vi "BMP180 Pull Raw Measurement.vi"(6 "Sensor Type":enum16{"Temp", "Pressure"}(ring), 8 "error in (no error)":errorcluster, 9 "BMP180 Config":T7={"I2C"={"Slave Address"=64, "Channel"=0}, "Mode"=enum."Ultra Low Power", "Cal Coefs"={"AC1"={"Addr:"=0, "Val:"=0}, "AC2"={"Addr:"=0, "Val:"=0}, "AC3"={"Addr:"=0, "Val:"=0}, "AC4"={"Addr:"=0, "Val:"=0}, "AC5"={"Addr:"=0, "Val:"=0}, "AC6"={"Addr:"=0, "Val:"=0}, "B1"={"Addr:"=0, "Val:"=0}, "B2"={"Addr:"=0, "Val:"=0}, "MB"={"Addr:"=0, "Val:"=0}, "MC"={"Addr:"=0, "Val:"=0}, "MD"={"Addr:"=0, "Val:"=0}}, "Online"=FALSE} {"I2C"."Slave Address" format="%.0x"; "Cal Coefs"."MD"."Val:" format="%04x"; "Cal Coefs"."MD"."Addr:" format="%02x"; "Cal Coefs"."MC"."Val:" format="%04x"; "Cal Coefs"."MC"."Addr:" format="%02x"; "Cal Coefs"."MB"."Val:" format="%04x"; "Cal Coefs"."MB"."Addr:" format="%02x"; "Cal Coefs"."B2"."Val:" format="%04x"; "Cal Coefs"."B2"."Addr:" format="%02x"; "Cal Coefs"."B1"."Val:" format="%04x"; "Cal Coefs"."B1"."Addr:" format="%02x"; "Cal Coefs"."AC6"."Val:" format="%04x"; "Cal Coefs"."AC6"."Addr:" format="%02x"; "Cal Coefs"."AC5"."Val:" format="%04x"; "Cal Coefs"."AC5"."Addr:" format="%02x"; "Cal Coefs"."AC4"."Val:" format="%04x"; "Cal Coefs"."AC4"."Addr:" format="%02x"; "Cal Coefs"."AC3"."Val:" format="%04x"; "Cal Coefs"."AC3"."Addr:" format="%02x"; "Cal Coefs"."AC2"."Val:" format="%04x"; "Cal Coefs"."AC2"."Addr:" format="%02x"; "Cal Coefs"."AC1"."Val:" format="%04x"; "Cal Coefs"."AC1"."Addr:" format="%02x"}, 11 "LINX Resource in":T1) -> (0 "error out":errorcluster, 2 "Raw Reading":i32, 3 "LINX Resource":T1)   [LabVIEW 2017]
uses:
  BMP180 Config Options.ctl
  <vilib>/MakerHub/LINX/Private/Type Defs/LINX Ref.ctl
  <vilib>/MakerHub/LINX/Private/Type Defs/Platform.ctl
  <vilib>/MakerHub/LINX/Private/Type Defs/Interface.ctl
  <vilib>/MakerHub/LINX/Private/Device/Type Defs/LINX Device Config.ctl
  <vilib>/MakerHub/LINX/Private/Device/Type Defs/TCP Config.ctl
  <vilib>/MakerHub/LINX/Private/Device/Type Defs/Channels.ctl
  <vilib>/MakerHub/LINX/LMH-LINX.lvlib
  <vilib>/MakerHub/LINX/Private/Device/Device.lvlib
panel:
  out "Data":u8[](array[numeric]) format="%.0x"
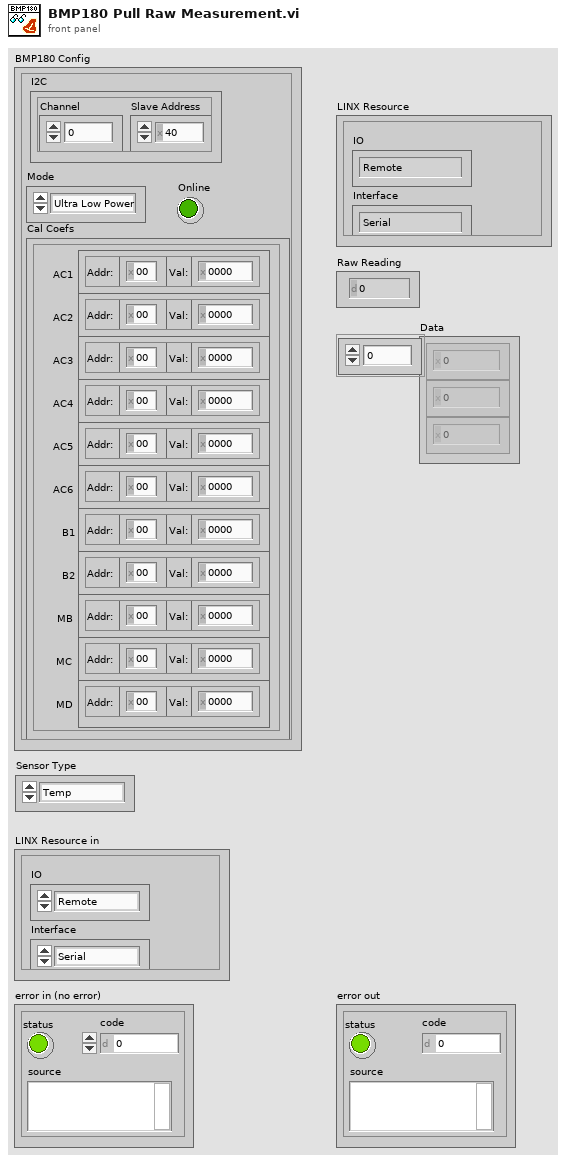
[diagram p1: front panel]
types:
  T1 = typedef "LMH-LINX.lvlib/LINX Ref.ctl" = cluster{"IO":T2, "Interface":T3, "LINX Device Config":T4}
  T2 = typedef "LMH-LINX.lvlib/Platform.ctl" = enum16{"Remote", "Local"}
  T3 = typedef "LMH-LINX.lvlib/Interface.ctl" = enum16{"Serial", "TCP"}
  T4 = typedef "LMH-LINX.lvlib/Device.lvlib/LINX Device Config.ctl" = cluster{"Interface":T3, "COM Port":refnum<visa-resource-name>, "TCP Configuration":T5, "Device Family":u8, "Device ID":u8, "Device Name":string, "TCP Ref":refnum<k5>, "Channels":T6}
  T5 = typedef "LMH-LINX.lvlib/Device.lvlib/TCP Config.ctl" = cluster{"IP Address":string, "Port":u16}
  T6 = typedef "LMH-LINX.lvlib/Channels.ctl" = cluster{"DI":u8[], "DO":u8[], "AI":u8[], "AO":u8[], "PWM":u8[], "QE":u8[], "UART":u8[], "I2C 2":u8[], "SPI":u8[], "CAN":u8[], "Servo":u8[], "AI Ref (V)":dbl, "AI Resolution (Bits)":u8, "AO Ref (V)":dbl, "AO Resolution (Bits)":u8}
  T7 = typedef "BMP180 Config Options.ctl" = cluster{"I2C":cluster{"Slave Address":u8, "Channel":u8}, "Mode":enum8{"Ultra Low Power", "Standard", "High Resolution", "Ultra High Resolution"}, "Cal Coefs":cluster{"AC1":cluster{"Addr:":u8, "Val:":u16}, "AC2":cluster{"Addr:":u8, "Val:":u16}, "AC3":cluster{"Addr:":u8, "Val:":u16}, "AC4":cluster{"Addr:":u8, "Val:":u16}, "AC5":cluster{"Addr:":u8, "Val:":u16}, "AC6":cluster{"Addr:":u8, "Val:":u16}, "B1":cluster{"Addr:":u8, "Val:":u16}, "B2":cluster{"Addr:":u8, "Val:":u16}, "MB":cluster{"Addr:":u8, "Val:":u16}, "MC":cluster{"Addr:":u8, "Val:":u16}, "MD":cluster{"Addr:":u8, "Val:":u16}}, "Online":bool}
  T8 = enum8{"Ultra Low Power", "Standard", "High Resolution", "Ultra High Resolution"}
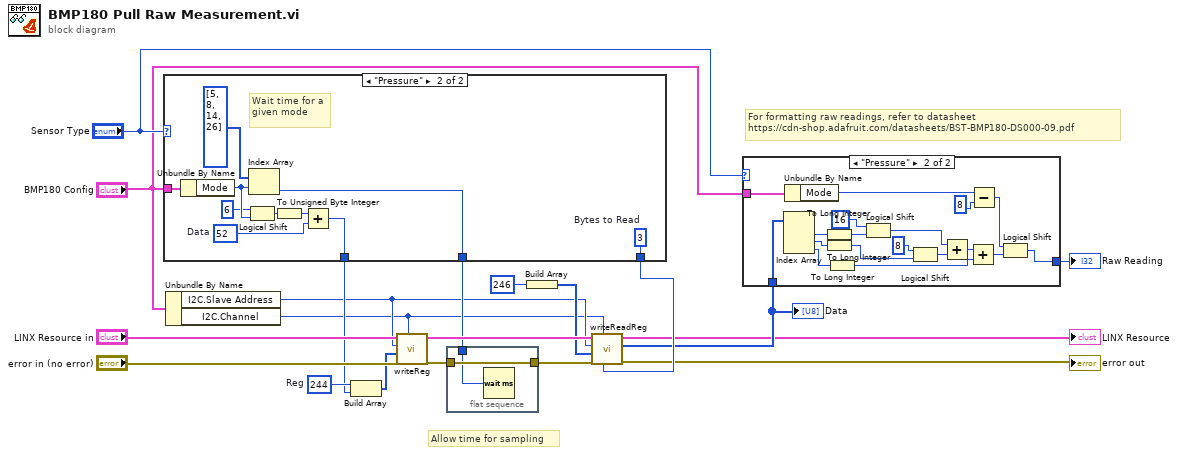
[diagram p0: block diagram]
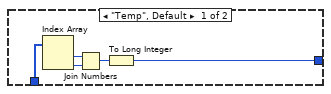
[diagram p2: hidden frame]
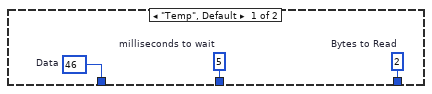
[diagram p3: hidden frame]
diagram:
  w14 = u8 244  # Reg
  # "For formatting raw readings, refer to datasheet\nhttps://cdn-shop.adafruit.com/datasheets/BST-BMP180-DS000-09.pdf"
  # "Allow time for sampling"
  n1 = case shown="\"Pressure\"" "Sensor Type" {
    tunnel: [w23 w31] -> w15
    tunnel: "BMP180 Config" -> [_ w33]
    tunnel: [w22 w25] -> w12
    tunnel: [w21 w24] -> w4
    frame "Temp", Default {
      w21 = u8 2  # Bytes to Read
      w22 = u8 46  # Data
      w23 = u32 5  # milliseconds to wait
    }
    frame "Pressure" {
      w24 = u8 3  # Bytes to Read
      w27 = u8 52  # Data
      # "Wait time for a given mode"
      n2 = Unbundle By Name(w33) -> ("Mode"=w30:T8)
      n3 = Logical Shift(y=i16 6, x=w30) -> (x << y=w28:u32)
      n4 = Index Array(array=u32[] [5, 8, 14, 26], index=w30) -> (element=w31:u32)
      n5 = To Unsigned Byte Integer(number=w28) -> (unsigned 8bit integer=w26:u8)
      n6 = Add(x=w26, y=w27) -> (x+y=w25:u8)
    }
  }
  n7 = Unbundle By Name("BMP180 Config") -> ("I2C.Slave Address"=w6:u8, "I2C.Channel"=w5:u8)
  n8 = Build Array(w14, w12) -> (w13:u8[])
  n9 = call "writeReg.vi"("I2C Channel"=w5, "error in"="error in (no error)", "Data"=w13, "I2C Slave Address"=w6, "LINX Resource in"="LINX Resource in") -> ("error out"=w18:errorcluster, "LINX Resource"=w19:T1)  [unwired: 5 in]
  n10 = flat-sequence {
    tunnel: [w35] -> w20
    tunnel: w18 -> [w35]
    tunnel: w15 -> [w34]
    frame #0 {
      n11 = Wait (ms)(milliseconds to wait=w34) -> ()  [unwired: 1 out]
    }
  }
  n12 = Build Array(u8 246 ("I2C Slave Address 2")) -> (w9:u8[])
  n13 = call "writeReadReg.vi"("Bytes To Read"=w4, "I2C Channel"=w5, "error in"=w20, "Data"=w9, "I2C Slave Address"=w6, "LINX Resource in"=w19) -> ("error out"=→"error out":errorcluster, "Bytes Read"=w3:u8[], "LINX Resource out"=→"LINX Resource":T1)  [unwired: 3 in]
  "Data" <- w3
  n14 = case shown="\"Pressure\"" "Sensor Type" {
    tunnel: w3 -> [w37 w58]
    tunnel: "BMP180 Config" -> [_ w57]
    tunnel: [w36 w41] -> w8
    frame "Temp", Default {
      n15 = Index Array(array=w37) -> (element #1=w40:u8, element #2=w39:u8)  [unwired: 2 in]
      n16 = Join Numbers(hi=w40, lo=w39) -> ((hi.lo)=w38:u16)
      n17 = To Long Integer(number=w38) -> (32bit integer=w36:i32)
    }
    frame "Pressure" {
      n18 = Index Array(array=w58) -> (element #1=w56:u8, element #2=w50:u8, element #3=w48:u8)  [unwired: 3 in]
      n19 = Unbundle By Name(w57) -> ("Mode"=w44:T8)
      n20 = To Long Integer(number=w56) -> (32bit integer=w55:i32)
      n21 = To Long Integer(number=w50) -> (32bit integer=w49:i32)
      n22 = To Long Integer(number=w48) -> (32bit integer=w47:i32)
      n23 = Logical Shift(y=i16 16, x=w55) -> (x << y=w52:i32)
      n24 = Logical Shift(y=i16 8, x=w49) -> (x << y=w53:i32)
      n25 = Add(x=w52, y=w53) -> (x+y=w46:i32)
      n26 = Add(x=w46, y=w47) -> (x+y=w45:i32)
      n27 = Subtract(x=w44, y=i16 8) -> (x-y=w42:i16)
      n28 = Logical Shift(y=w42, x=w45) -> (x << y=w41:i32)
    }
  }
  "Raw Reading" <- w8
